vi "VI Ref to Queue.vi"(4 "VI Refnum":refnum<vi>) -> (1 "queue out":refnum<queue>)   [LabVIEW 2013]
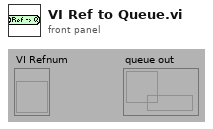
[diagram p1: front panel]
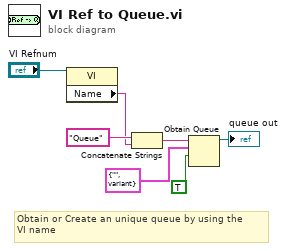
[diagram p0: block diagram]
diagram:
  # "Obtain or Create an unique queue by using the \nVI name"
  n1 = property class="VI"(reference="VI Refnum") -> ("Name"=w3:string)  [unwired: 1 in, 2 out]
  n2 = Concatenate Strings("Queue" ("string"), w3) -> (w5:string)
  n3 = Obtain Queue(name (unnamed)=w5, element data type=cluster{string, "Variant":variant} {"", "Variant"=variant}, create if not found? (T)=TRUE) -> (queue out=→"queue out":refnum<queue>)  [unwired: 2 in, 2 out]
